vi "New Operations.vi"(8 "error in (no error)":errorcluster caption="entrée d'erreur (pas d'erreur)", 10 "initial dictionary (empty)":cluster{"key":variant, "value":variant}[](array[cluster]), 11 "Operations en entrée":refnum<class "Operations.lvclass"> caption="DNL_LabVIEW Object in") -> (0 "error out":errorcluster caption="sortie d'erreur", 3 "Operations en sortie":refnum<class "Operations.lvclass"> caption="DNL_LabVIEW Object out")   [LabVIEW 2012, in "Operations.lvclass"]
uses:
  Operations.lvclass
  Operations.lvclass/Operations.ctl
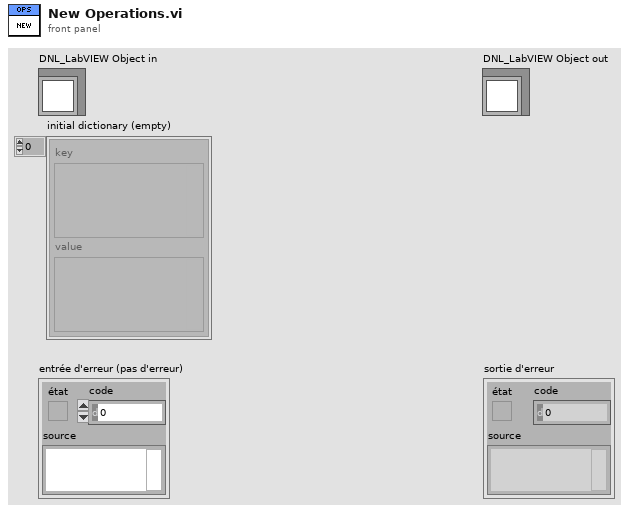
[diagram p1: front panel]
types:
  T1 = typedef "Dictionary Object RefNum__ogtk.ctl" = refnum<k1>
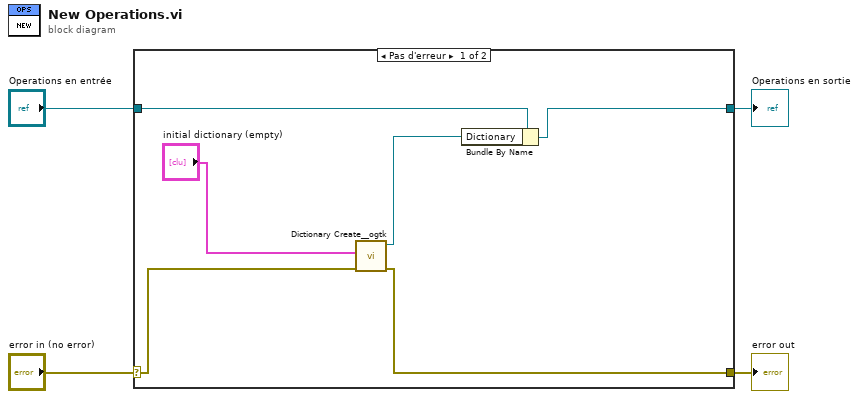
[diagram p0: block diagram]
diagram:
  n1 = case shown="Pas d'erreur" "error in (no error)" {
    selector: "error in (no error)" -> [w6 w12]
    tunnel: [w7 w12] -> w3
    tunnel: [w9 w11] -> w1
    tunnel: "Operations en entrée" -> [w10 w11]
    frame No Error {
      n2 = call <userlib>:"Dictionary Create__ogtk.vi"("error in (no error)"=w6, "initial dictionary (empty)"="initial dictionary (empty)") -> ("error out"=w7:errorcluster, "dictionary out"=w8:T1)  [unwired: 8 in]
      n3 = Bundle By Name(cluster=w10, "Dictionary"=w8) -> (w9:refnum<class "Operations.lvclass">)
    }
    frame Error {
    }
  }
  "error out" <- w3
  "Operations en sortie" <- w1
